vi "example2.vi"() -> ()   [LabVIEW 2018, in "LV-Julia_ZMQ-Roundtrip_lib.lvlib"]
uses:
  LV-Julia_ZMQ-Roundtrip_lib.lvlib
  Commands v2.ctl
panel:
  out "error now":errorcluster
  out "error out":errorcluster
  out "server response":string
  in  "data to send":string="hello"
  in  "stop":bool
  in  "milliseconds to wait":u32=1000
  in  "Julia ZMQ server file name":string="ZMQ-testserver2.jl"
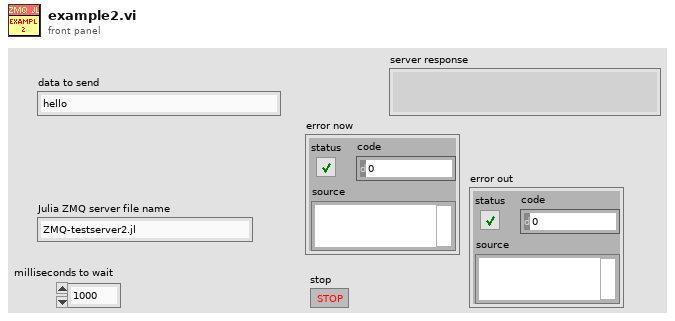
[diagram p1: front panel]
types:
  T1 = typedef "LV-Julia_ZMQ-Roundtrip_lib.lvlib/Commands v2.ctl" = enum16{"Start Jl-server & Init LV-client", "Send request & Get response ", "Stop Jl-server & Cleanup LV-client", "Cleanup LV-client", "Start Jl-server", "Stop Jl-server", "Init LV-Client", "Cleanup LV-Client", "(not allowed)", "Set LV Client state", "Set Jl Server state"}
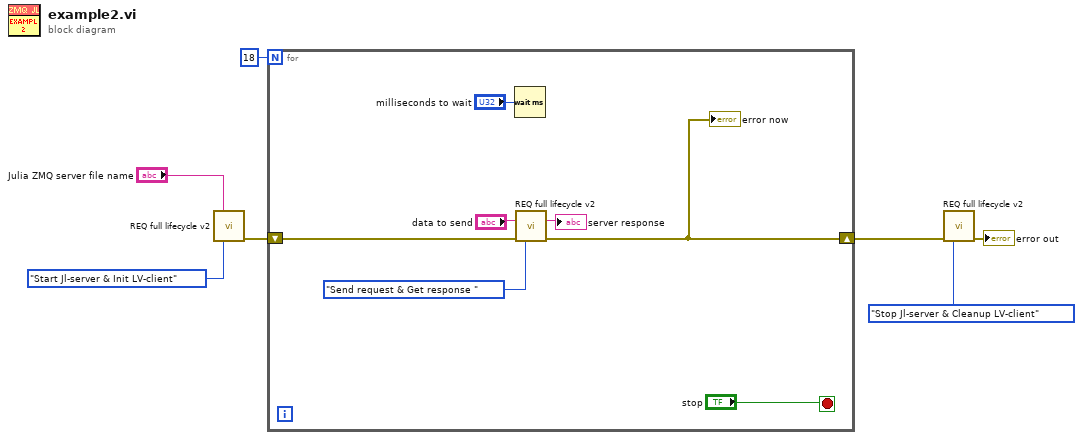
[diagram p0: block diagram]
diagram:
  n1 = call "REQ full lifecycle v2.vi"("Julia ZMQ server file name"="Julia ZMQ server file name", "command"=Commands_v2."Start Jl-server & Init LV-client") -> ("error out"=w6:errorcluster)  [unwired: 10 in, 3 out]
  n2 = for {
    N: 18 -> [_]
    shift-right: [w12] -> w5
    shift-left: w6 -> [w13]
    stop <- "stop" stop-if-true
    n3 = Wait (ms)(milliseconds to wait="milliseconds to wait") -> ()  [unwired: 1 out]
    n4 = call "REQ full lifecycle v2.vi"("data to send"="data to send", "error in"=w13, "command"=Commands_v2."Send request & Get response ") -> ("server response"=→"server response":string, "error out"=w12:errorcluster)  [unwired: 9 in, 2 out]
    "error now" <- w12
  }
  n5 = call "REQ full lifecycle v2.vi"("error in"=w5, "command"=Commands_v2."Stop Jl-server & Cleanup LV-client") -> ("error out"=→"error out":errorcluster)  [unwired: 10 in, 3 out]
